vi "svfa_Map Parameters for DZT.vi"(8 "fs":dbl format="%.2f", 9 "stop frequency":dbl format="%.2f", 10 "start frequency":dbl format="%.2f", 11 "Block Size":i32) -> (0 "df":dbl format="%.2f", 1 "f0":dbl format="%.2f", 2 "output length":i32, 3 "FFT length":i32, 5 "start index":i32, 7 "M":i32)   [LabVIEW 2017]
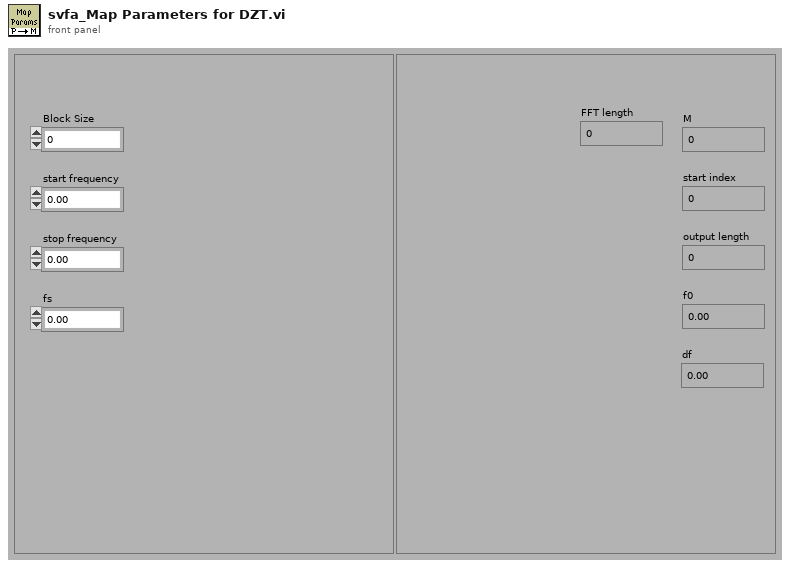
[diagram p1: front panel]
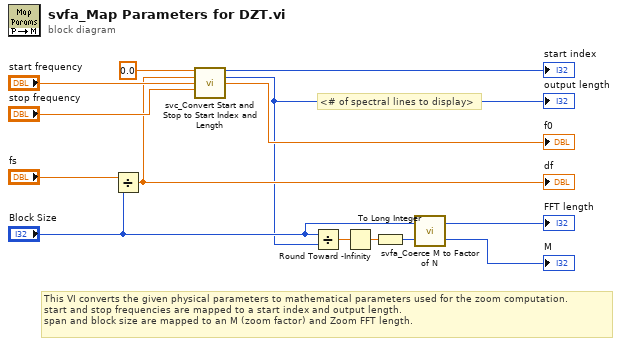
[diagram p0: block diagram]
diagram:
  # "<# of spectral lines to display>"
  # "This VI converts the given physical parameters to mathematical parameters used for the zoom computation.\nstart and stop frequencies are mapped to a start index and output length.\nspan and block size are mapped to an M (zoom factor) and Zoom FFT length."
  n1 = Divide(x="fs", y="Block Size") -> (x/y=w5:dbl)
  "df" <- w5
  n2 = call <vilib>:"svc_Convert Start and Stop to Start Index and Length.vi"("f0"=0.0, "df"=w5, "start frequency"="start frequency", "stop frequency"="stop frequency") -> ("start index"=→"start index":i32, "band length"=w1:i32, "f0 out"=→"f0":dbl)  [unwired: 8 in, 1 out]
  "output length" <- w1
  n3 = Divide(x="Block Size", y=w1) -> (x/y=w14:dbl)
  n4 = Round Toward -Infinity ("Round To -Infinity")(1:w14) -> (0:w13:dbl)
  n5 = To Long Integer(number=w13) -> (32bit integer=w12:i32)
  n6 = call <vilib>:"svfa_Coerce M to Factor of N.vi"("M"=w12, "Block Size"="Block Size") -> ("Coerced M"=→"M":i32, "Zoom FFT Size"=→"FFT length":i32)
